vi "ARGBSetChannelValueCore.vi"(7 "Channel":T1, 8 "error in (no error)":errorcluster, 10 "Value":u8, 11 "Src in":T2) -> (0 "error out":errorcluster)   [LabVIEW 2020, in "image.lvlib"]
uses:
  image.lvlib
  ARGB Image.ctl
  ARGBChannels.ctl
  common/common.lvlib
  common/bin/gartoolkit_32-1.dll
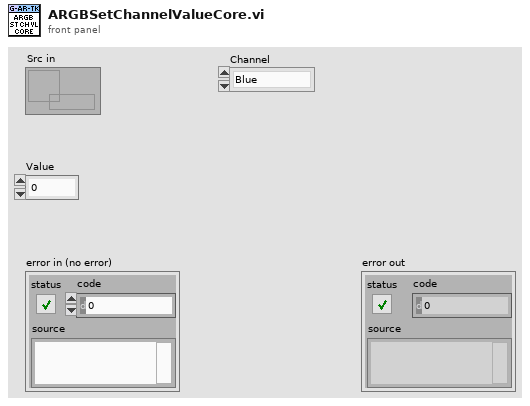
[diagram p1: front panel]
types:
  T1 = typedef "image.lvlib/ARGBChannels.ctl" = enum8{"Blue", "Green", "Red", "Alpha"}
  T2 = typedef "image.lvlib/ARGB Image.ctl" = refnum<data-value>
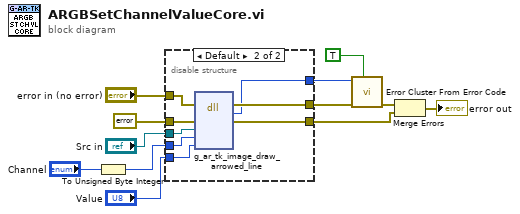
[diagram p0: block diagram]
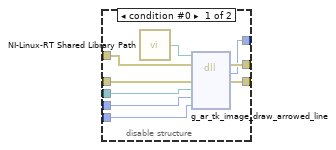
[diagram p2: hidden frame]
diagram:
  n1 = To Unsigned Byte Integer(number="Channel") -> (unsigned 8bit integer=w7:u8)
  n2 = disable-structure shown="Default" {
    disable-tunnel: "error in (no error)" -> [w21 w29]
    disable-tunnel: errorcluster {"status"=FALSE, "code"=0, "source"=""} ("error constant") -> [w20 w28]
    disable-tunnel: "Src in" -> [w19 w27]
    disable-tunnel: w7 -> [w18 w26]
    disable-tunnel: "Value" -> [w17 w25]
    disable-tunnel: [w16 w24] -> w5
    disable-tunnel: [w15 w23] -> w4
    disable-tunnel: [w14 w22] -> w3
    frame condition #0 {
      n3 = call "NI-Linux-RT Shared Library Path.vi"() -> ("Path"=w13:path)
      n4 = dll-call lib="?" fn="g_ar_tk_image_draw_arrowed_line"(path in=w13, error in=w21, "error_cluster"=w20, "EDVR src"=w19, "Channel"=w18, "Value"=w17) -> (error out=w16:errorcluster, "MgErr"=w15:i32, "error_cluster"=w14:errorcluster)  [unwired: 4 in, 1 out]
    }
    frame condition #1 (active) {
      n5 = dll-call lib="C:/serenial/lib/g-augmented-reality-toolkit/LabVIEW/common/bin/gartoolkit_*-1.*" fn="g_ar_tk_image_draw_arrowed_line"(error in=w29, "error_cluster"=w28, "EDVR src"=w27, "Channel"=w26, "Value"=w25) -> (error out=w24:errorcluster, "MgErr"=w23:i32, "error_cluster"=w22:errorcluster)  [unwired: 5 in, 1 out]
    }
  }
  n6 = call <vilib>:"Error Cluster From Error Code.vi"("show call chain? (False)"=TRUE, "error in (no error)"=w5, "error code (0)"=w4) -> ("error out"=w11:errorcluster)  [unwired: 6 in]
  n7 = Merge Errors(w11, w3) -> (→"error out":errorcluster)
